vi "dfd_nMAC_CircAddNwEn.vi"(1 "len":fxp<+,16,16>, 2 "idxIn":fxp<+,16,16>, 3 "Enable":bool, 4 "step":fxp<+,16,16>) -> (6 "opWrap?":bool, 7 "idxOut":fxp<+,16,16>)   [LabVIEW 2017]
doc: "opWrap is NOT cleared even if Enable==False."
uses:
  <vilib>/rvi/FXPMathLib/basic elements/FxpAddSub/XNode/nifxpmath_AddSub.xnode
  <vilib>/rvi/FXPMathLib/sim/FxpSim.dll
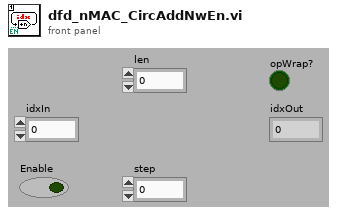
[diagram p1: front panel]
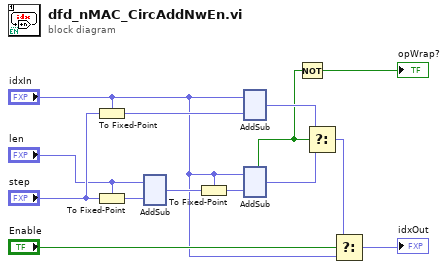
[diagram p0: block diagram]
diagram:
  n1 = To Fixed-Point(fixed-point type="idxIn", number="step") -> (fixed-point=w3:fxp<+,16,16>)
  n2 = To Fixed-Point(fixed-point type="len", number="step") -> (fixed-point=w5:fxp<+,16,16>)
  n3 = xnode "AddSub"("x"="len", "y"=w5) -> ("s"=w6:fxp<+,16,16>)  [unwired: 1 out]
  n4 = To Fixed-Point(fixed-point type="idxIn", number=w6) -> (fixed-point=w2:fxp<+,16,16>)
  n5 = xnode "AddSub"("x"="idxIn", "y"=w3) -> ("s"=w14:fxp<+,16,16>)  [unwired: 1 out]
  n6 = xnode "AddSub"("x"="idxIn", "y"=w2) -> ("s"=w13:fxp<+,16,16>, "borrow-out"=w12:bool)
  n7 = Not(x=w12) -> (.not. x?=→"opWrap?":bool)
  n8 = Select(t=w14, s=w12, f=w13) -> (s? t:f=w10:fxp<+,16,16>)
  n9 = Select(t=w10, s="Enable", f="idxIn") -> (s? t:f=→"idxOut":fxp<+,16,16>)
